vi "Calculate Jogwheel Delta.vi"(10 "New Value":i32, 11 "Old Value":i32) -> (3 "Delta Value":i32)   [LabVIEW 2019, in "User Interface.lvlib"]
doc: "Calculate the delta value from two jogwheel values. Delta value will be shortest distance between old and new values, including sign (clockwise is positive, anti-clockwise is negative)."
uses:
  User Interface.lvlib
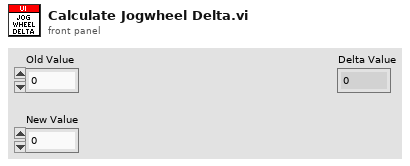
[diagram p1: front panel]
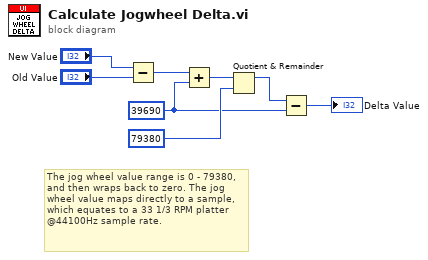
[diagram p0: block diagram]
diagram:
  w4 = 39690 ("y")
  # "The jog wheel value range is 0 - 79380, and then wraps back to zero. The jog wheel value maps directly to a sample, which equates to a 33 1/3 RPM platter @44100Hz sample rate."
  n1 = Subtract(x="New Value", y="Old Value") -> (x-y=w8:i32)
  n2 = Add(x=w8, y=w4) -> (x+y=w7:i32)
  n3 = Quotient & Remainder(x=w7, y=79380) -> (x-y*floor(x/y)=w5:i32)  [unwired: 1 out]
  n4 = Subtract(x=w5, y=w4) -> (x-y=→"Delta Value":i32)
